vi "Read Action.vi"(8 "error in (no error)":errorcluster, 11 "Background Loop Msg in":refnum<class "Background Loop Msg.lvclass">) -> (0 "error out":errorcluster, 2 "Action":T1, 3 "Background Loop Msg out":refnum<class "Background Loop Msg.lvclass">)   [LabVIEW 2021, in "Background Loop Msg.lvclass"]
uses:
  Background Loop Msg.lvclass
  Worker Actor/Background Loop Action.ctl
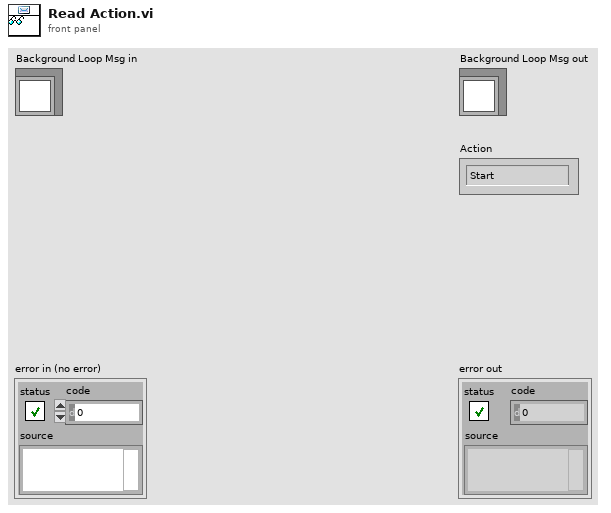
[diagram p1: front panel]
types:
  T1 = typedef "Background Loop Action.ctl" = enum16{"Start", "Continue", "Stop"}
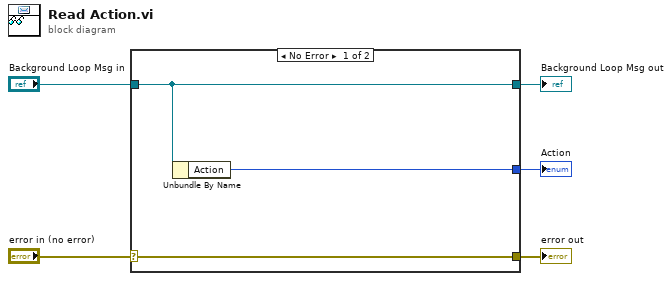
[diagram p0: block diagram]
diagram:
  n1 = case shown="No Error" "error in (no error)" {
    selector: "error in (no error)" -> [w8 w9]
    tunnel: [w8 w9] -> w4
    tunnel: [w7 w10] -> w2
    tunnel: "Background Loop Msg in" -> [w7 w10]
    tunnel: [w6 _] -> w1
    frame No Error {
      n2 = Unbundle By Name(w7) -> ("Action"=w6:T1)
    }
    frame Error {
    }
  }
  "error out" <- w4
  "Background Loop Msg out" <- w2
  "Action" <- w1
